vi "Get Registered Claims.vi"(0 "JSONWebToken in":refnum<class "JSONWebToken.lvclass">, 11 "error in (no error)":errorcluster) -> (3 "payload (JSON)":string, 4 "JSONWebToken out":refnum<class "JSONWebToken.lvclass">, 8 "registered claims":T1, 15 "error out":errorcluster)   [LabVIEW 2017, in "JSONWebToken.lvclass"]
doc: "<B>Registered Claim Names</B>\n\nClaim Names are registered in the IANA \"JSON Web Token Claims\" registry established by Section 10.1. \n\nNone of the claims returned are intended to be mandatory to use or implement in all cases, but rather they provide a starting point for a set of useful, interoperable claims. Applications using JWTs should define which specific claims they use and when they are required or optional. All the names are short because a core goal of JWTs is for the representation to be compact.\n\nThe JSON representation of the claims is exposed as an optional output at the top of this VI for access to the full claim set."
uses:
  JSONWebToken.lvclass
  JWT registered Claims -- cluster.ctl
  JSONWebToken.lvclass/JSONWebToken.ctl
  cbe48e1a-5b77-4676-a575-71ac047a5681.vi
  <vilib>/addons/_JKI.lib/Serialization/JSON/JKI JSON Serialization.lvlib
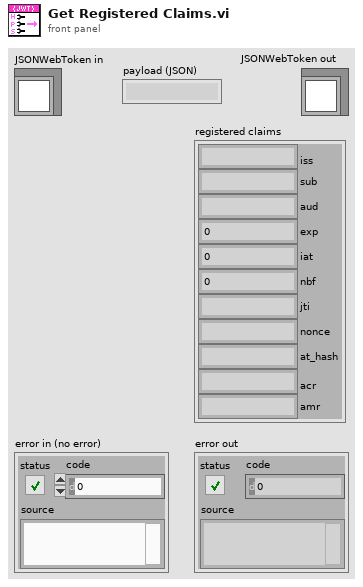
[diagram p1: front panel]
types:
  T1 = typedef "JSONWebToken.lvclass/JWT registered Claims -- cluster.ctl" = cluster{"iss":string, "sub":string, "aud":string, "exp":i32, "iat":i32, "nbf":i32, "jti":string, "nonce":string, "at_hash":string, "acr":string, "amr":string}
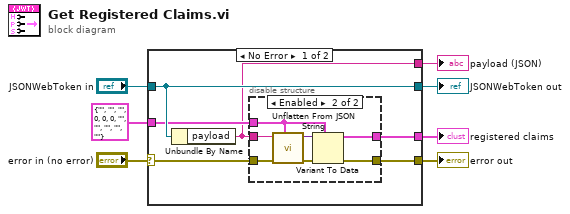
[diagram p0: block diagram]
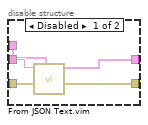
[diagram p2: hidden frame]
diagram:
  n1 = case shown="No Error" "error in (no error)" {
    selector: "error in (no error)" -> [w9 w26]
    tunnel: "JSONWebToken in" -> [w13 w27]
    tunnel: T1 {"iss"="", "sub"="", "aud"="", "exp"=0, "iat"=0, "nbf"=0, "jti"="", "nonce"="", "at_hash"="", "acr"="", "amr"=""} -> [w12 _]
    tunnel: [w13 w27] -> w4
    tunnel: [w11 _] -> w3
    tunnel: [w10 w26] -> w2
    tunnel: [w8 _] -> w1
    frame No Error {
      n2 = Unbundle By Name(w13) -> ("payload"=w8:string)
      n3 = disable-structure shown="Enabled" {
        disable-tunnel: w8 -> [w18 w25]
        disable-tunnel: w12 -> [w17 w20]
        disable-tunnel: w9 -> [w16 w19]
        disable-tunnel: [w15 w21] -> w10
        disable-tunnel: [w14 w22] -> w11
        frame Disabled {
          n4 = call "From JSON Text.vim"("Data Type and Default Value"=w17, "error in (no error)"=w16, "JSON"=w18) -> ("error out"=w15:errorcluster, "Data out"=w14:T1)  [unwired: 7 in]
        }
        frame Enabled {
          n5 = call <vilib>:"Unflatten From JSON String.vi"("Type and Defaults"=w20, "error in"=w19, "JSON String"=w25) -> ("error out"=w24:errorcluster, "Variant"=w23:variant)  [unwired: 7 in]
          n6 = Variant To Data(error in=w24, type=w20, Variant=w23) -> (data=w22:T1, error out=w21:errorcluster)
        }
      }
    }
    frame Error {
    }
  }
  "JSONWebToken out" <- w4
  "registered claims" <- w3
  "error out" <- w2
  "payload (JSON)" <- w1
